vi "Read Before Trigger Delay.vi"(0 "RedPitaya TCP Connection in":refnum<k5>, 3 "# Samples Before Trigger Delay":u16, 5 "error in":errorcluster, 8 "Channel #":u16(ring)=1 items=["Channel 1"=1, "Channel 2"=2], 12 "timeout ms (2000)":i32=2000) -> (14 "RedPitaya TCP Connection out":refnum<k5>, 16 "Measurement Array":dbl[](array[numeric]), 19 "error out":errorcluster)   [LabVIEW 2010, in "RedPitaya.lvlib"]
doc: "Read m samples before trigger delay. Trigger delay by default is set to zero (in samples or in seconds). If trigger delay is set to zero it will read m samples before trigger."
uses:
  RedPitaya.lvlib
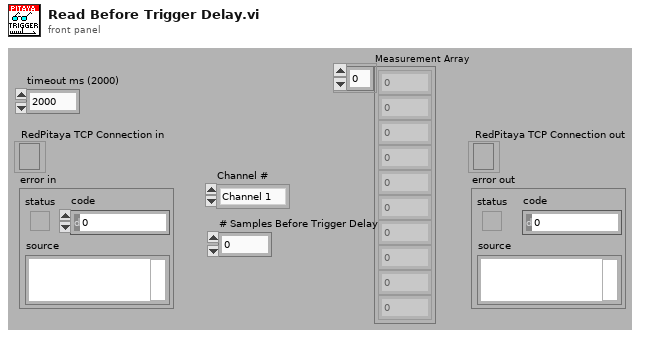
[diagram p1: front panel]
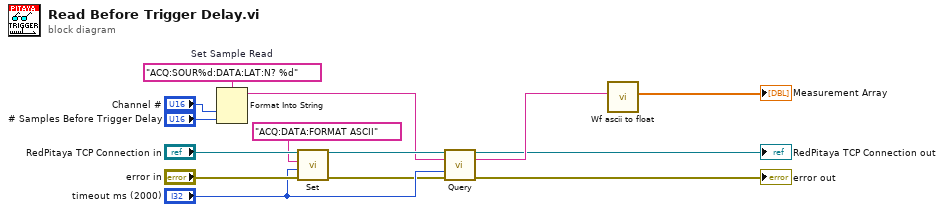
[diagram p0: block diagram]
diagram:
  w14 = "ACQ:SOUR%d:DATA:LAT:N? %d"  # Set Sample Read
  n1 = Format Into String(format string=w14, "Channel #", "# Samples Before Trigger Delay") -> (resulting string=w6:string)  [unwired: 2 in, 1 out]
  n2 = call "Set.vi"("error in"="error in", "timeout ms (2000)"="timeout ms (2000)", "SCPI Message"="ACQ:DATA:FORMAT ASCII", "RedPitaya connection in"="RedPitaya TCP Connection in") -> ("error out"=w4:errorcluster, "RedPitaya connection out"=w7:refnum<k5>)  [unwired: 5 in, 1 out]
  n3 = call "Query.vi"("RedPitaya connection in"=w7, "SCPI Query"=w6, "timeout ms (2000)"="timeout ms (2000)", "error in"=w4) -> ("RedPitaya connection out"=→"RedPitaya TCP Connection out":refnum<k5>, "data out"=w2:string, "error out"=→"error out":errorcluster)  [unwired: 9 in]
  n4 = call "Wf ascii to float.vi"("String array"=w2) -> ("Array out"=→"Measurement Array":dbl[])  [unwired: 10 in]
